vi "Initialize Subpanels.vi"(8 "error in (no error)":errorcluster) -> (0 "error out":errorcluster)   [LabVIEW 2018, in "Main.lvlib"]
uses:
  ADM/Main.lvlib
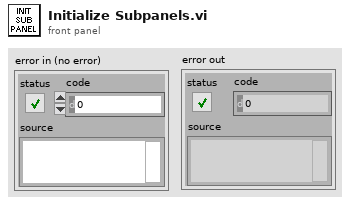
[diagram p1: front panel]
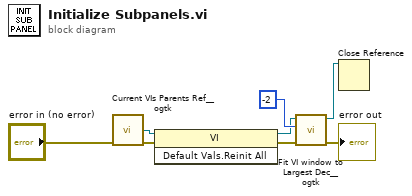
[diagram p0: block diagram]
diagram:
  n1 = call <userlib>:"Current VIs Parents Ref__ogtk.vi"() -> ("Calling VI's Reference"=w5:refnum<vi>)  [unwired: 2 in]
  n2 = invoke class="VI" method="Default Vals.Reinit All"(reference=w5, error in="error in (no error)") -> (reference out=w2:refnum<vi>, error out=w6:errorcluster)  [unwired: 1 in, 1 out]
  n3 = call <userlib>:"Fit VI window to Largest Dec__ogtk.vi"("error in (no error)"=w6, "border spacing (2 px)"=-2, "VI Ref (calling VI)"=w2) -> ("error out"=→"error out":errorcluster, "dup VI Ref"=w1:refnum<vi>)  [unwired: 3 in]
  n4 = Close Reference(reference=w1) -> ()  [unwired: 1 in, 1 out]
